vi "Compare Timestamp Index.vi"(10 "Index Timestamp":u64, 11 "Log Timestamp":string="08/22/2023\t16:45:51") -> (3 "Past":bool)   [LabVIEW 2021, in "CIFLogs.lvlib"]
uses:
  CIFLogs.lvlib
  CIFClocks/CIFClocks.lvlib
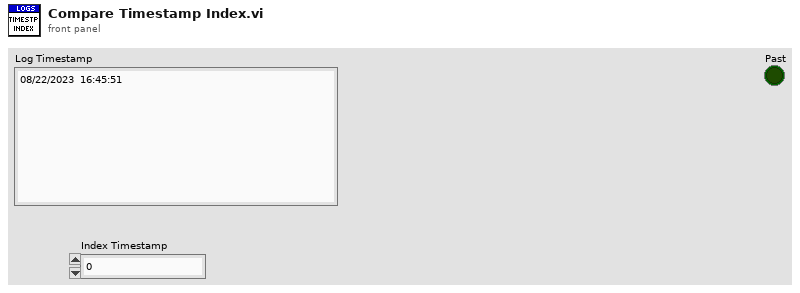
[diagram p1: front panel]
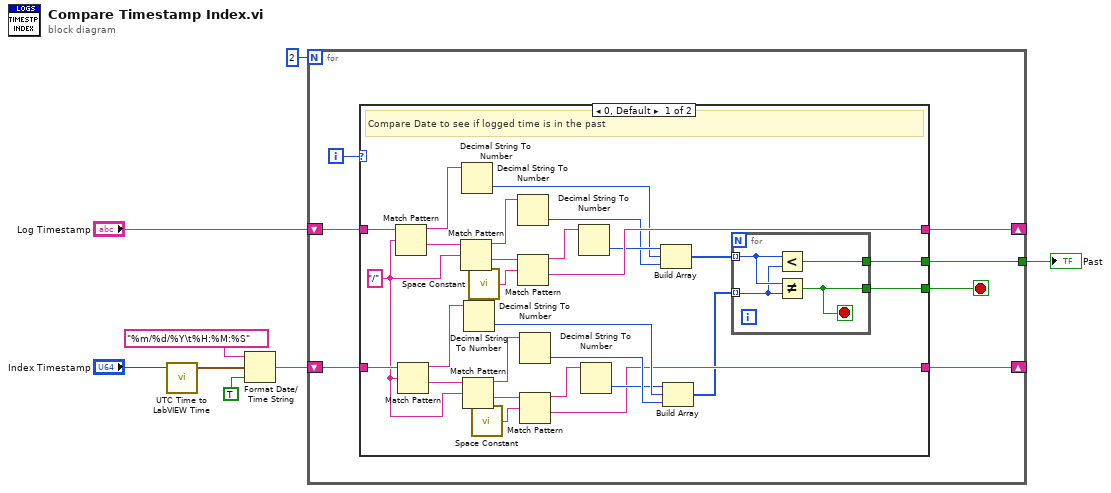
[diagram p0: block diagram]
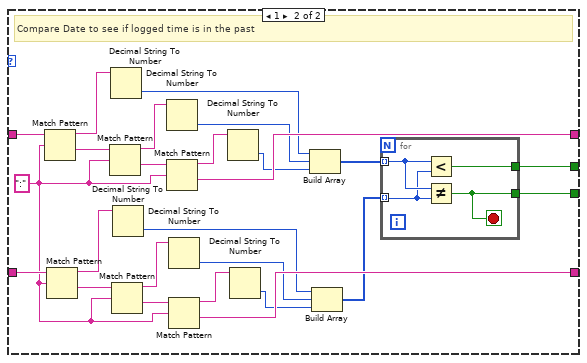
[diagram p2: hidden frame]
diagram:
  n1 = call "UTC Time to LabVIEW Time.vi"("UTC Time (ns)"="Index Timestamp") -> ("LabVIEW Time (s)"=w7:timestamp)  [unwired: 4 in]
  n2 = Format Date/Time String(time format string (%c)="%m/%d/%Y\t%H:%M:%S", seconds (now)=w7, UTC format=TRUE) -> (date/time string=w4:string)
  n3 = for {
    N: 2 -> [_]
    shift-right: [w12] -> _
    shift-left: "Log Timestamp" -> [w14]
    shift-right: [w11] -> _
    shift-left: w4 -> [w13]
    tunnel: [w10] -> w3
    i -> [w15]
    stop <- w9 stop-if-true
    n4 = case shown="0, Default" w15 {
      tunnel: w14 -> [w42 w71]
      tunnel: w13 -> [w24 w59]
      tunnel: [w36 w65] -> w12
      tunnel: [w23 w58] -> w11
      tunnel: [w20 w55] -> w9
      tunnel: [w19 w54] -> w10
      frame 0, Default {
        w18 = "/"
        # "Compare Date to see if logged time is in the past"
        n5 = Match Pattern(string=w42, regular expression=w18) -> (before substring=w39:string, after substring=w41:string)  [unwired: 1 in, 2 out]
        n6 = Match Pattern(string=w24, regular expression=w18) -> (before substring=w27:string, after substring=w25:string)  [unwired: 1 in, 2 out]
        n7 = Match Pattern(string=w41, regular expression=w18) -> (before substring=w38:string, after substring=w40:string)  [unwired: 1 in, 2 out]
        n8 = Decimal String To Number(string=w39) -> (number=w34:i32)  [unwired: 2 in, 1 out]
        n9 = Match Pattern(string=w25, regular expression=w18) -> (before substring=w28:string, after substring=w26:string)  [unwired: 1 in, 2 out]
        n10 = Decimal String To Number(string=w27) -> (number=w31:i32)  [unwired: 2 in, 1 out]
        n11 = call <vilib>:"Space Constant.vi"() -> ("String"=w17:string)
        n12 = call <vilib>:"Space Constant.vi"() -> ("String"=w16:string)
        n13 = Decimal String To Number(string=w38) -> (number=w33:i32)  [unwired: 2 in, 1 out]
        n14 = Match Pattern(string=w40, regular expression=w17) -> (before substring=w37:string, after substring=w36:string)  [unwired: 1 in, 2 out]
        n15 = Decimal String To Number(string=w28) -> (number=w32:i32)  [unwired: 2 in, 1 out]
        n16 = Match Pattern(string=w26, regular expression=w16) -> (before substring=w29:string, after substring=w23:string)  [unwired: 1 in, 2 out]
        n17 = Decimal String To Number(string=w37) -> (number=w35:i32)  [unwired: 2 in, 1 out]
        n18 = Decimal String To Number(string=w29) -> (number=w30:i32)  [unwired: 2 in, 1 out]
        n19 = Build Array(w35, w34, w33) -> (w22:i32[])
        n20 = Build Array(w30, w31, w32) -> (w21:i32[])
        n21 = for {
          tunnel: w22 -> [w45] mode=indexing
          tunnel: w21 -> [w44] mode=indexing
          tunnel: [w46] -> w20
          tunnel: [w43] -> w19
          stop <- w46 stop-if-true
          n22 = Less?(x=w45, y=w44) -> (x < y?=w43:bool)
          n23 = Not Equal?(x=w45, y=w44) -> (x != y?=w46:bool)
        }
      }
      frame 1 {
        w53 = ":"
        # "Compare Date to see if logged time is in the past"
        n24 = Match Pattern(string=w71, regular expression=w53) -> (before substring=w68:string, after substring=w70:string)  [unwired: 1 in, 2 out]
        n25 = Match Pattern(string=w59, regular expression=w53) -> (before substring=w62:string, after substring=w60:string)  [unwired: 1 in, 2 out]
        n26 = Match Pattern(string=w70, regular expression=w53) -> (before substring=w67:string, after substring=w69:string)  [unwired: 1 in, 2 out]
        n27 = Decimal String To Number(string=w68) -> (number=w50:i32)  [unwired: 2 in, 1 out]
        n28 = Match Pattern(string=w60, regular expression=w53) -> (before substring=w63:string, after substring=w61:string)  [unwired: 1 in, 2 out]
        n29 = Decimal String To Number(string=w62) -> (number=w49:i32)  [unwired: 2 in, 1 out]
        n30 = Decimal String To Number(string=w67) -> (number=w51:i32)  [unwired: 2 in, 1 out]
        n31 = Match Pattern(string=w69, regular expression=w53) -> (before substring=w66:string, after substring=w65:string)  [unwired: 1 in, 2 out]
        n32 = Decimal String To Number(string=w63) -> (number=w48:i32)  [unwired: 2 in, 1 out]
        n33 = Match Pattern(string=w61, regular expression=w53) -> (before substring=w64:string, after substring=w58:string)  [unwired: 1 in, 2 out]
        n34 = Decimal String To Number(string=w66) -> (number=w52:i32)  [unwired: 2 in, 1 out]
        n35 = Decimal String To Number(string=w64) -> (number=w47:i32)  [unwired: 2 in, 1 out]
        n36 = Build Array(w50, w51, w52) -> (w57:i32[])
        n37 = Build Array(w49, w48, w47) -> (w56:i32[])
        n38 = for {
          tunnel: w57 -> [w74] mode=indexing
          tunnel: w56 -> [w73] mode=indexing
          tunnel: [w75] -> w55
          tunnel: [w72] -> w54
          stop <- w75 stop-if-true
          n39 = Less?(x=w74, y=w73) -> (x < y?=w72:bool)
          n40 = Not Equal?(x=w74, y=w73) -> (x != y?=w75:bool)
        }
      }
    }
  }
  "Past" <- w3
